vi "filter.filter.other.vi"(11 "filter.data in":T1 {"memory.command"."order.slot.value"."Quantity" format="%016x"; "memory.command"."order.slot.value"."OrderId" format="%016x"; "memory.command"."ticker.slot.value"."Symbol" format="%016x"; "Scratch"."OrderId" format="%016x"}) -> (3 "filter.data out":T1 {"memory.command"."order.slot.value"."Quantity" format="%016x"; "memory.command"."order.slot.value"."OrderId" format="%016x"; "memory.command"."ticker.slot.value"."Symbol" format="%016x"; "Scratch"."OrderId" format="%016x"})   [LabVIEW 2022 SP3]
uses:
  filter.data.ctl
  filter.states.ctl
  filter.debug.ctl
  filter.debug.slot.ctl
  filter.data.scratch.ctl
  arty/orderbook/orderbook.command.ctl
  arty/orderbook/orderbook.command.type.ctl
  filter.memory.command.ctl
  ticker.slot.ctl
  order.slot.ctl
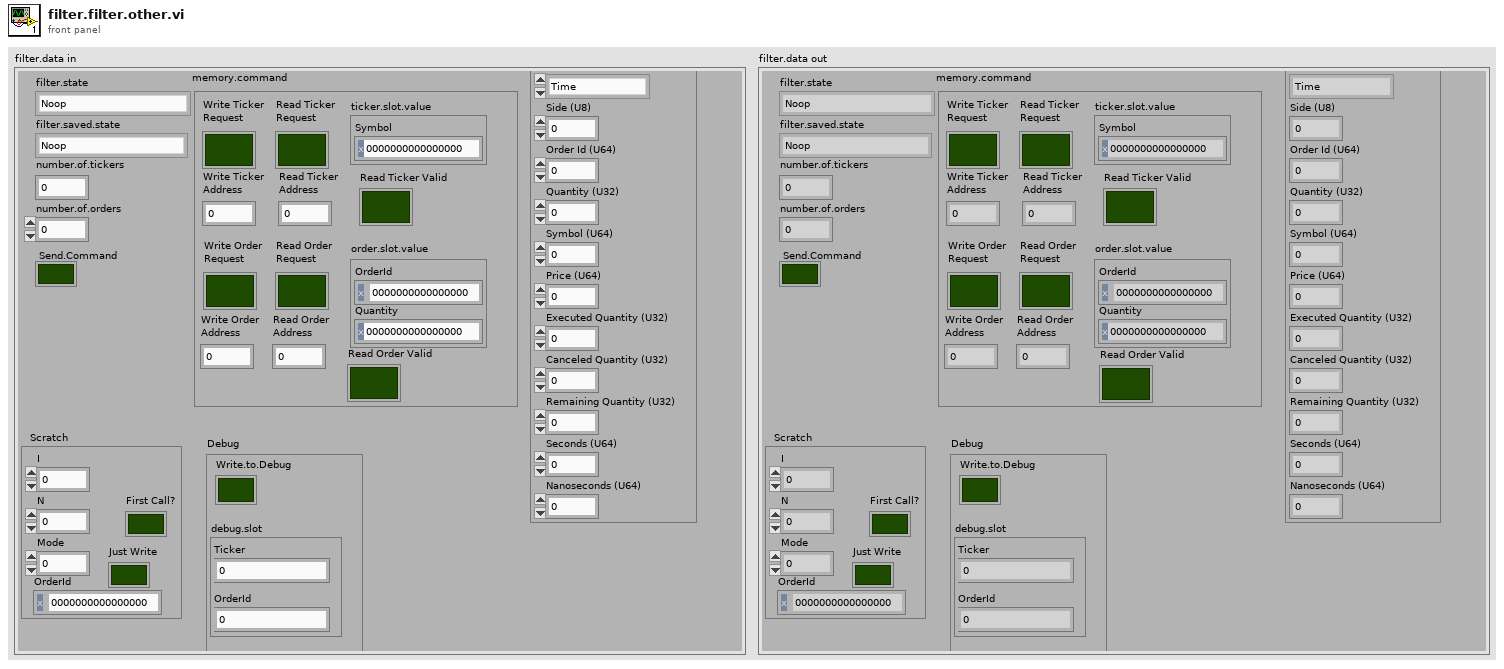
[diagram p1: front panel]
types:
  T1 = typedef "filter.data.ctl" = cluster{"filter.state":T2, "Debug":T3, "number.of.tickers":u32, "number.of.orders":u32, "filter.saved.state":T2, "Scratch":T5, "OrderBook.Command":T6, "Send.Command":bool, "memory.command":T8}
  T2 = typedef "filter.states.ctl" = enum16{"Noop", "Reset", "Debug", "Configuration", "Wait.for.Command", "Filter.Add", "Filter.Other", "Insert.Order", "Delete Order"}
  T3 = typedef "filter.debug.ctl" = cluster{"Write.to.Debug":bool, "debug.slot":T4}
  T4 = typedef "filter.debug.slot.ctl" = cluster{"Ticker":u64, "OrderId":u64}
  T5 = typedef "filter.data.scratch.ctl" = cluster{"I":u32, "N":u32, "Mode":u32, "OrderId":u64, "First Call?":bool, "Just Write":bool}
  T6 = typedef "orderbook.command.ctl" = cluster{"OrderBook Command.Type":T7, "Side (U8)":u8, "Order Id (U64)":u64, "Quantity (U32)":u32, "Symbol (U64)":u64, "Price (U64)":u64, "Executed Quantity (U32)":u32, "Canceled Quantity (U32)":u32, "Remaining Quantity (U32)":u32, "Seconds (U64)":u64, "Nanoseconds (U64)":u64}
  T7 = typedef "orderbook.command.type.ctl" = enum16{"Time", "AddOrder", "OrderExecuted", "OrderExecutedAtPrice", "ReduceSize", "ModifyOrder", "DeleteOrder", "Get.All.Orders", "Get.Top"}
  T8 = typedef "filter.memory.command.ctl" = cluster{"ticker.slot.value":T9, "order.slot.value":T10, "Write Ticker\nAddress":u32, "Write Ticker\nRequest":bool, "Read Ticker\nRequest":bool, "Read Ticker\nAddress":u32, "Read Ticker Valid":bool, "Write Order\nAddress":u32, "Write Order\nRequest":bool, "Read Order\nRequest":bool, "Read Order\nAddress":u32, "Read Order Valid":bool}
  T9 = typedef "ticker.slot.ctl" = cluster{"Symbol":u64}
  T10 = typedef "order.slot.ctl" = cluster{"OrderId":u64, "Quantity":u64}
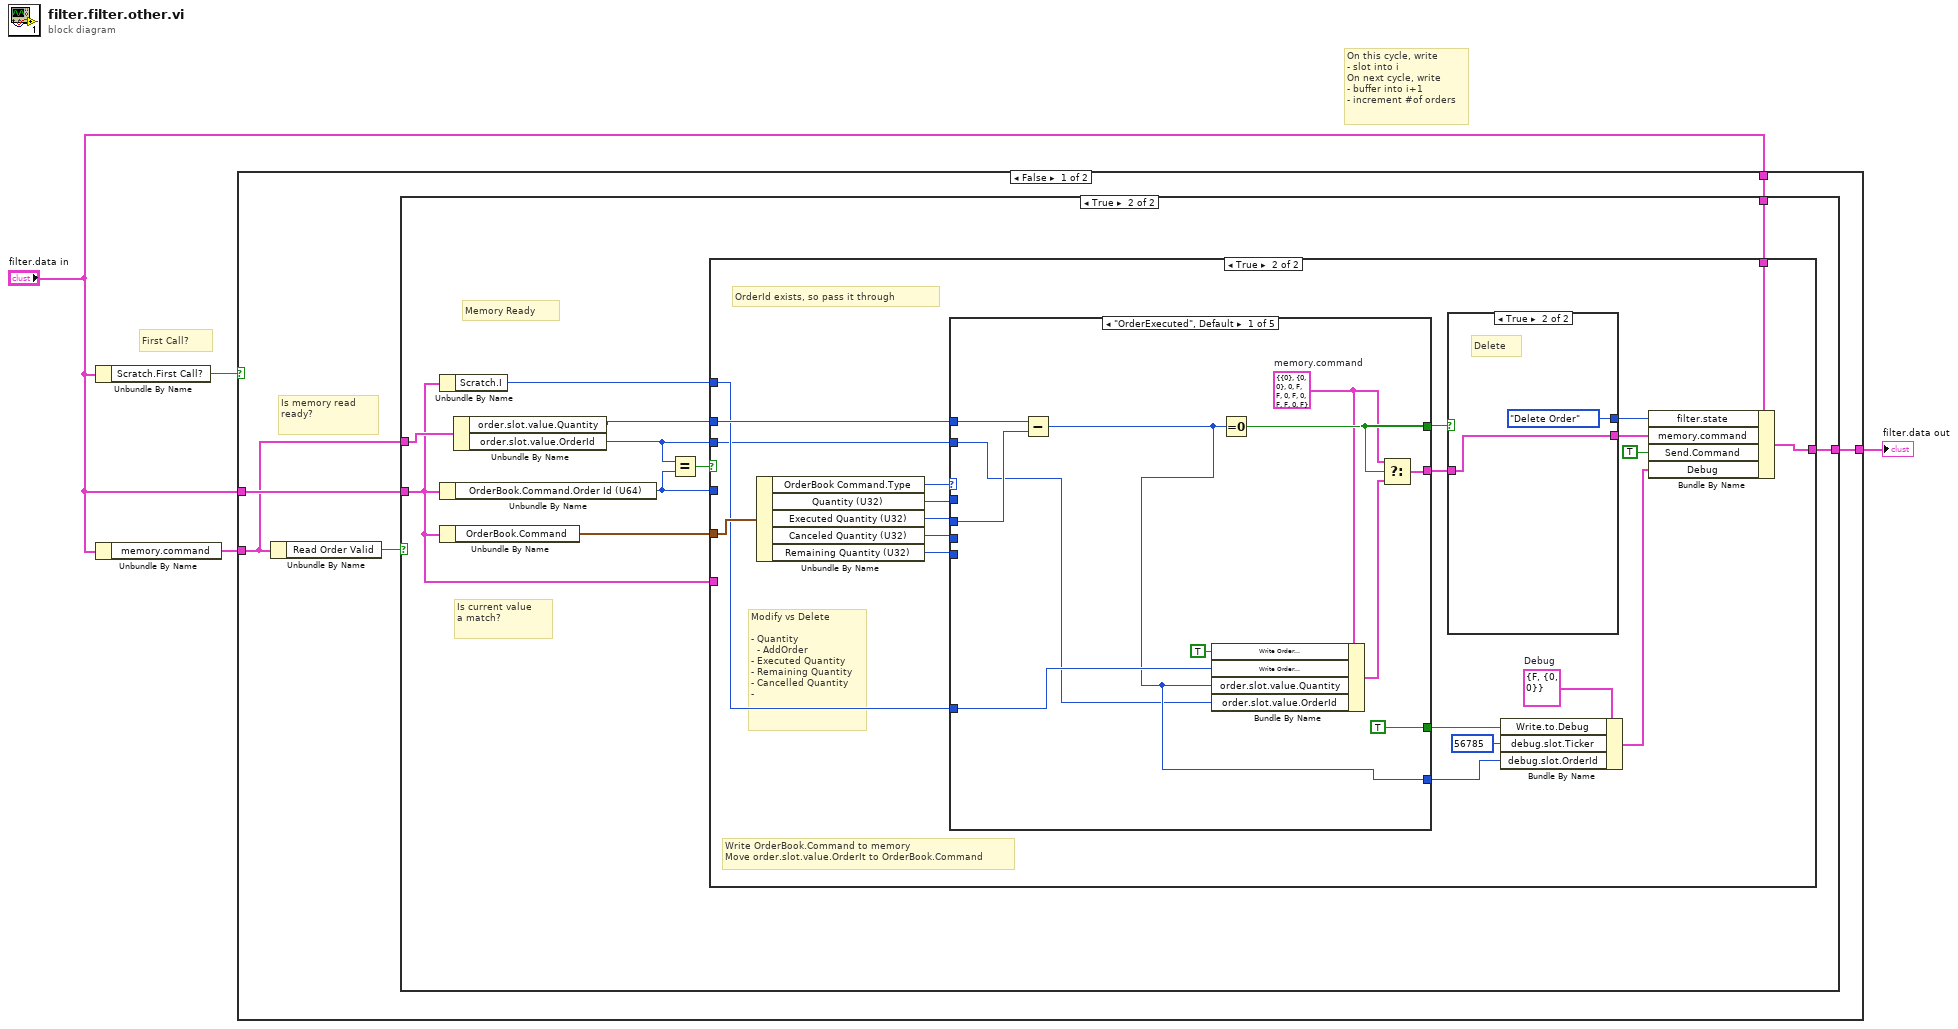
[diagram p0: block diagram]
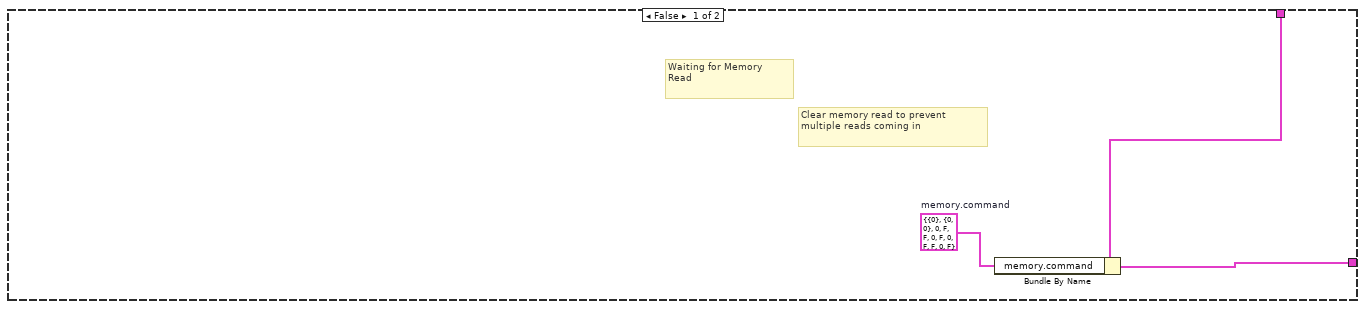
[diagram p2: hidden frame]
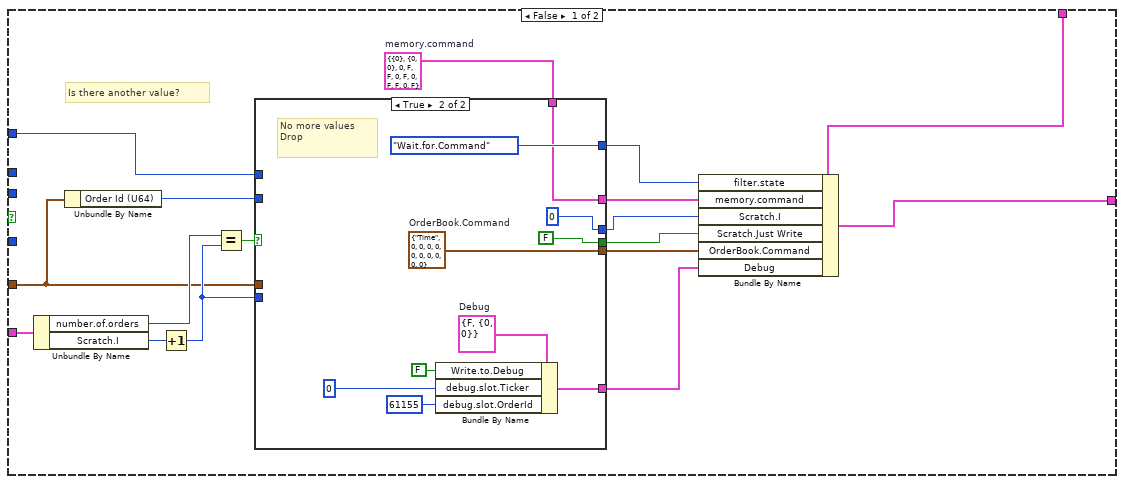
[diagram p3: hidden frame]
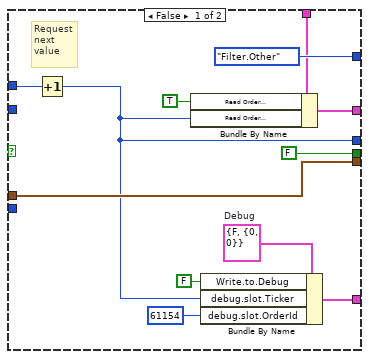
[diagram p4: hidden frame]
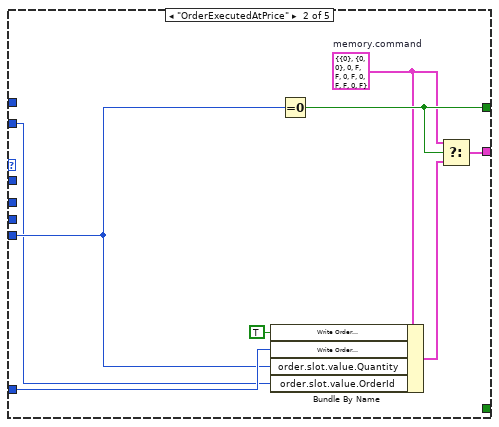
[diagram p5: hidden frame]
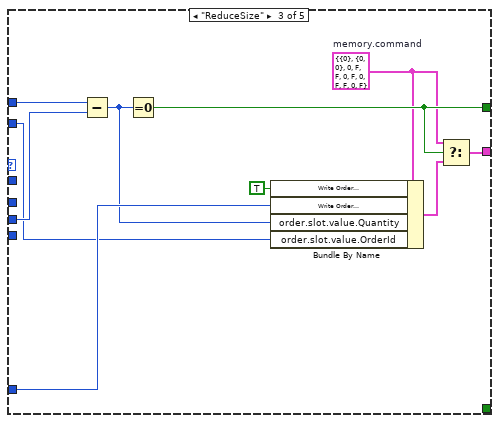
[diagram p6: hidden frame]
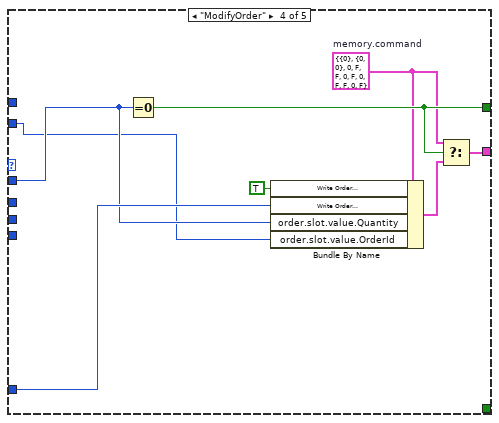
[diagram p7: hidden frame]
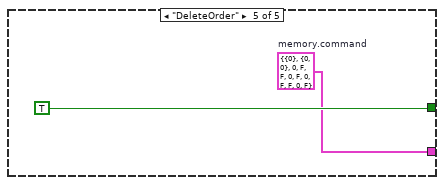
[diagram p8: hidden frame]
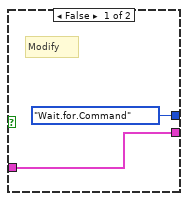
[diagram p9: hidden frame]
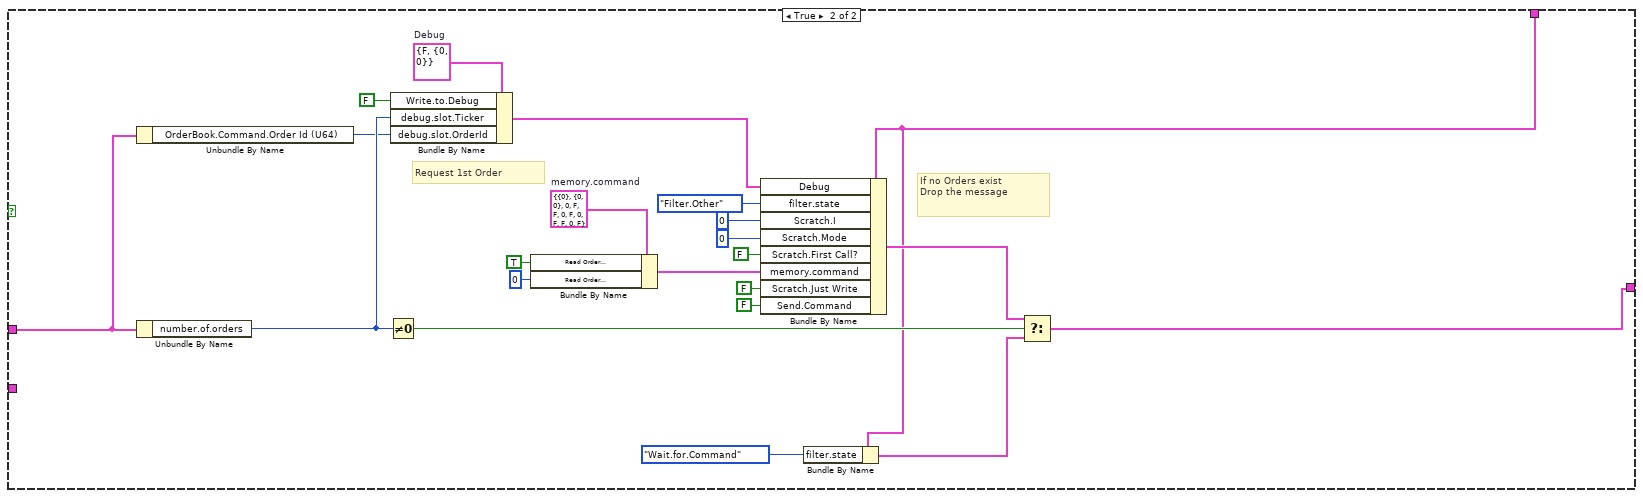
[diagram p10: hidden frame]
diagram:
  # "On this cycle, write\n- slot into i\nOn next cycle, write\n- buffer into i+1\n- increment #of orders"
  # "First Call?"
  n1 = Unbundle By Name("filter.data in") -> ("Scratch.First Call?"=w1:bool)
  n2 = Unbundle By Name("filter.data in") -> ("memory.command"=w3:T8)
  n3 = case shown="False" w1 {
    tunnel: "filter.data in" -> [w8 w127]
    tunnel: [w9 w128] -> w2
    tunnel: w3 -> [w6 _]
    tunnel: "filter.data in" -> [w7 w129]
    frame False {
      # "Is memory read\nready?"
      n4 = Unbundle By Name(w6) -> ("Read Order Valid"=w5:bool)
      n5 = case shown="True" w5 {
        tunnel: [w10 w20] -> w9
        tunnel: w8 -> [w12 w21]
        tunnel: w7 -> [_ w19]
        tunnel: w6 -> [_ w22]
        frame False {
          w11 = T8 {"ticker.slot.value"={"Symbol"=0}, "order.slot.value"={"OrderId"=0, "Quantity"=0}, "Write Ticker\nAddress"=0, "Write Ticker\nRequest"=FALSE, "Read Ticker\nRequest"=FALSE, "Read Ticker\nAddress"=0, "Read Ticker Valid"=FALSE, "Write Order\nAddress"=0, "Write Order\nRequest"=FALSE, "Read Order\nRequest"=FALSE, "Read Order\nAddress"=0, "Read Order Valid"=FALSE}  # memory.command
          # "Clear memory read to prevent\nmultiple reads coming in"
          # "Waiting for Memory\nRead"
          n6 = Bundle By Name(cluster=w12, "memory.command"=w11) -> (w10:T1)
        }
        frame True {
          # "Is current value\na match?"
          # "Memory Ready"
          n7 = Unbundle By Name(w19) -> ("Scratch.I"=w14:u32)
          n8 = Unbundle By Name(w19) -> ("OrderBook.Command.Order Id (U64)"=w15:u64)
          n9 = Unbundle By Name(w19) -> ("OrderBook.Command"=w17:T6)
          n10 = Unbundle By Name(w22) -> ("order.slot.value.Quantity"=w13:u64, "order.slot.value.OrderId"=w16:u64)
          n11 = Equal?(x=w16, y=w15) -> (x = y?=w18:bool)
          n12 = case shown="True" w18 {
            tunnel: w21 -> [w38 w82]
            tunnel: [w39 w80] -> w20
            tunnel: w17 -> [w24 w79]
            tunnel: w19 -> [w37 _]
            tunnel: w16 -> [_ w62]
            tunnel: w14 -> [w29 w70]
            tunnel: w15 -> [_ _]
            tunnel: w13 -> [_ w74]
            frame False {
              w31 = T8 {"ticker.slot.value"={"Symbol"=0}, "order.slot.value"={"OrderId"=0, "Quantity"=0}, "Write Ticker\nAddress"=0, "Write Ticker\nRequest"=FALSE, "Read Ticker\nRequest"=FALSE, "Read Ticker\nAddress"=0, "Read Ticker Valid"=FALSE, "Write Order\nAddress"=0, "Write Order\nRequest"=FALSE, "Read Order\nRequest"=FALSE, "Read Order\nAddress"=0, "Read Order Valid"=FALSE}  # memory.command
              # "Is there another value?"
              n13 = Unbundle By Name(w37) -> ("number.of.orders"=w28:u32, "Scratch.I"=w36:u32)
              n14 = Unbundle By Name(w24) -> ("Order Id (U64)"=w30:u64)
              n15 = Increment(x=w36) -> (x+1=w33:u32)
              n16 = Equal?(x=w28, y=w33) -> (x = y?=w34:bool)
              n17 = case shown="True" w34 {
                tunnel: [w51 w53] -> w35
                tunnel: w33 -> [_ _]
                tunnel: [filter.states."Filter.Other" ("filter.state") filter.states."Wait.for.Command" ("filter.state")] -> w32
                tunnel: w31 -> [w48 w53]
                tunnel: w30 -> [_ _]
                tunnel: w29 -> [w41 _]
                tunnel: [w40 u32 0] -> w27
                tunnel: [FALSE ("Scratch.Just Write") FALSE ("Scratch.Just Write")] -> w26
                tunnel: [w46 w58] -> w25
                tunnel: w24 -> [w46 _]
                tunnel: [w44 w56] -> w23
                frame False {
                  w45 = T3 {"Write.to.Debug"=FALSE, "debug.slot"={"Ticker"=0, "OrderId"=0}}  # Debug
                  # "Request\nnext\nvalue"
                  n18 = Increment(x=w41) -> (x+1=w40:u32)
                  n19 = Bundle By Name(cluster=w48, "Read Order\nRequest"=TRUE ("Read.Request"), "Read Order\nAddress"=w40) -> (w51:T8)
                  n20 = Bundle By Name(cluster=w45, "Write.to.Debug"=FALSE, "debug.slot.Ticker"=w40, "debug.slot.OrderId"=u64 61154) -> (w44:T3)
                }
                frame True {
                  w57 = T3 {"Write.to.Debug"=FALSE, "debug.slot"={"Ticker"=0, "OrderId"=0}}  # Debug
                  w58 = T6 {"OrderBook Command.Type"=enum."Time", "Side (U8)"=0, "Order Id (U64)"=0, "Quantity (U32)"=0, "Symbol (U64)"=0, "Price (U64)"=0, "Executed Quantity (U32)"=0, "Canceled Quantity (U32)"=0, "Remaining Quantity (U32)"=0, "Seconds (U64)"=0, "Nanoseconds (U64)"=0}  # OrderBook.Command
                  # "No more values\nDrop"
                  n21 = Bundle By Name(cluster=w57, "Write.to.Debug"=FALSE, "debug.slot.Ticker"=u64 0, "debug.slot.OrderId"=u64 61155) -> (w56:T3)
                }
              }
              n22 = Bundle By Name(cluster=w38, "filter.state"=w32, "memory.command"=w35, "Scratch.I"=w27, "Scratch.Just Write"=w26, "OrderBook.Command"=w25, "Debug"=w23) -> (w39:T1)
            }
            frame True {
              w77 = T3 {"Write.to.Debug"=FALSE, "debug.slot"={"Ticker"=0, "OrderId"=0}}  # Debug
              # "Modify vs Delete\n\n- Quantity\n  - AddOrder\n- Executed Quantity\n- Remaining Quantity\n- Cancelled Quantity\n-"
              # "Write OrderBook.Command to memory\nMove order.slot.value.OrderIt to OrderBook.Command"
              # "OrderId exists, so pass it through"
              n23 = Unbundle By Name(w79) -> ("OrderBook Command.Type"=w75:T7, "Quantity (U32)"=w68:u32, "Executed Quantity (U32)"=w65:u32, "Canceled Quantity (U32)"=w66:u32, "Remaining Quantity (U32)"=w67:u32)
              n24 = case shown="\"OrderExecuted\", Default" w75 {
                tunnel: w74 -> [w93 _ w111 _ _]
                tunnel: w68 -> [_ _ _ w113 _]
                tunnel: [w91 w100 w109 w118 TRUE] -> w73
                tunnel: [w89 w98 w107 w116 w120] -> w72
                tunnel: w70 -> [w87 w96 w105 w114 _]
                tunnel: w67 -> [_ w95 _ _ _]
                tunnel: w66 -> [_ _ w103 _ _]
                tunnel: w65 -> [w86 _ _ _ _]
                tunnel: [TRUE ("Write.to.Debug") _ _ _ _] -> w64
                tunnel: [w84 _ _ _ _] -> w63
                tunnel: w62 -> [w83 w94 w102 w112 _]
                frame "OrderExecuted", Default {
                  w88 = T8 {"ticker.slot.value"={"Symbol"=0}, "order.slot.value"={"OrderId"=0, "Quantity"=0}, "Write Ticker\nAddress"=0, "Write Ticker\nRequest"=FALSE, "Read Ticker\nRequest"=FALSE, "Read Ticker\nAddress"=0, "Read Ticker Valid"=FALSE, "Write Order\nAddress"=0, "Write Order\nRequest"=FALSE, "Read Order\nRequest"=FALSE, "Read Order\nAddress"=0, "Read Order Valid"=FALSE}  # memory.command
                  n25 = Subtract(x=w93, y=w86) -> (x-y=w84:u64)
                  n26 = Bundle By Name(cluster=w88, "Write Order\nRequest"=TRUE ("Read.Request"), "Write Order\nAddress"=w87, "order.slot.value.Quantity"=w84, "order.slot.value.OrderId"=w83) -> (w90:T8)
                  n27 = Equal To 0?(x=w84) -> (x = 0?=w91:bool)
                  n28 = Select(t=w88, s=w91, f=w90) -> (s? t:f=w89:T8)
                }
                frame "OrderExecutedAtPrice" {
                  w97 = T8 {"ticker.slot.value"={"Symbol"=0}, "order.slot.value"={"OrderId"=0, "Quantity"=0}, "Write Ticker\nAddress"=0, "Write Ticker\nRequest"=FALSE, "Read Ticker\nRequest"=FALSE, "Read Ticker\nAddress"=0, "Read Ticker Valid"=FALSE, "Write Order\nAddress"=0, "Write Order\nRequest"=FALSE, "Read Order\nRequest"=FALSE, "Read Order\nAddress"=0, "Read Order Valid"=FALSE}  # memory.command
                  n29 = Bundle By Name(cluster=w97, "Write Order\nRequest"=TRUE ("Read.Request"), "Write Order\nAddress"=w96, "order.slot.value.Quantity"=w95, "order.slot.value.OrderId"=w94) -> (w99:T8)
                  n30 = Equal To 0?(x=w95) -> (x = 0?=w100:bool)
                  n31 = Select(t=w97, s=w100, f=w99) -> (s? t:f=w98:T8)
                }
                frame "ReduceSize" {
                  w106 = T8 {"ticker.slot.value"={"Symbol"=0}, "order.slot.value"={"OrderId"=0, "Quantity"=0}, "Write Ticker\nAddress"=0, "Write Ticker\nRequest"=FALSE, "Read Ticker\nRequest"=FALSE, "Read Ticker\nAddress"=0, "Read Ticker Valid"=FALSE, "Write Order\nAddress"=0, "Write Order\nRequest"=FALSE, "Read Order\nRequest"=FALSE, "Read Order\nAddress"=0, "Read Order Valid"=FALSE}  # memory.command
                  n32 = Subtract(x=w111, y=w103) -> (x-y=w104:u64)
                  n33 = Equal To 0?(x=w104) -> (x = 0?=w109:bool)
                  n34 = Bundle By Name(cluster=w106, "Write Order\nRequest"=TRUE ("Read.Request"), "Write Order\nAddress"=w105, "order.slot.value.Quantity"=w104, "order.slot.value.OrderId"=w102) -> (w108:T8)
                  n35 = Select(t=w106, s=w109, f=w108) -> (s? t:f=w107:T8)
                }
                frame "ModifyOrder" {
                  w115 = T8 {"ticker.slot.value"={"Symbol"=0}, "order.slot.value"={"OrderId"=0, "Quantity"=0}, "Write Ticker\nAddress"=0, "Write Ticker\nRequest"=FALSE, "Read Ticker\nRequest"=FALSE, "Read Ticker\nAddress"=0, "Read Ticker Valid"=FALSE, "Write Order\nAddress"=0, "Write Order\nRequest"=FALSE, "Read Order\nRequest"=FALSE, "Read Order\nAddress"=0, "Read Order Valid"=FALSE}  # memory.command
                  n36 = Equal To 0?(x=w113) -> (x = 0?=w118:bool)
                  n37 = Bundle By Name(cluster=w115, "Write Order\nRequest"=TRUE ("Read.Request"), "Write Order\nAddress"=w114, "order.slot.value.Quantity"=w113, "order.slot.value.OrderId"=w112) -> (w117:T8)
                  n38 = Select(t=w115, s=w118, f=w117) -> (s? t:f=w116:T8)
                }
                frame "DeleteOrder" {
                  w120 = T8 {"ticker.slot.value"={"Symbol"=0}, "order.slot.value"={"OrderId"=0, "Quantity"=0}, "Write Ticker\nAddress"=0, "Write Ticker\nRequest"=FALSE, "Read Ticker\nRequest"=FALSE, "Read Ticker\nAddress"=0, "Read Ticker Valid"=FALSE, "Write Order\nAddress"=0, "Write Order\nRequest"=FALSE, "Read Order\nRequest"=FALSE, "Read Order\nAddress"=0, "Read Order Valid"=FALSE}  # memory.command
                }
              }
              n39 = case shown="True" w73 {
                tunnel: [filter.states."Wait.for.Command" ("filter.state") filter.states."Delete Order" ("filter.state")] -> w81
                tunnel: [w122 w124] -> w71
                tunnel: w72 -> [w122 w124]
                frame False {
                  # "Modify"
                }
                frame True {
                  # "Delete"
                }
              }
              n40 = Bundle By Name(cluster=w77, "Write.to.Debug"=w64, "debug.slot.Ticker"=u64 56785, "debug.slot.OrderId"=w63) -> (w69:T3)
              n41 = Bundle By Name(cluster=w82, "filter.state"=w81, "memory.command"=w71, "Send.Command"=TRUE, "Debug"=w69) -> (w80:T1)
            }
          }
        }
      }
    }
    frame True {
      w136 = T3 {"Write.to.Debug"=FALSE, "debug.slot"={"Ticker"=0, "OrderId"=0}}  # Debug
      w146 = T8 {"ticker.slot.value"={"Symbol"=0}, "order.slot.value"={"OrderId"=0, "Quantity"=0}, "Write Ticker\nAddress"=0, "Write Ticker\nRequest"=FALSE, "Read Ticker\nRequest"=FALSE, "Read Ticker\nAddress"=0, "Read Ticker Valid"=FALSE, "Write Order\nAddress"=0, "Write Order\nRequest"=FALSE, "Read Order\nRequest"=FALSE, "Read Order\nAddress"=0, "Read Order Valid"=FALSE}  # memory.command
      # "If no Orders exist\nDrop the message"
      # "Request 1st Order"
      n42 = Unbundle By Name(w129) -> ("OrderBook.Command.Order Id (U64)"=w132:u64)
      n43 = Unbundle By Name(w129) -> ("number.of.orders"=w133:u32)
      n44 = Not Equal To 0?(x=w133) -> (x != 0?=w131:bool)
      n45 = Bundle By Name(cluster=w136, "Write.to.Debug"=FALSE, "debug.slot.Ticker"=w133, "debug.slot.OrderId"=w132) -> (w134:T3)
      n46 = Bundle By Name(cluster=w146, "Read Order\nRequest"=TRUE ("Read.Request"), "Read Order\nAddress"=u32 0 ("Read Order\nAddress")) -> (w141:T8)
      n47 = Bundle By Name(cluster=w127, "Debug"=w134, "filter.state"=filter.states."Filter.Other", "Scratch.I"=u32 0, "Scratch.Mode"=u32 0, "Scratch.First Call?"=FALSE, "memory.command"=w141, "Scratch.Just Write"=FALSE, "Send.Command"=FALSE) -> (w140:T1)
      n48 = Bundle By Name(cluster=w127, "filter.state"=filter.states."Wait.for.Command") -> (w139:T1)
      n49 = Select(t=w140, s=w131, f=w139) -> (s? t:f=w128:T1)
    }
  }
  "filter.data out" <- w2
